vi "Compound_arithmetics.vi"() -> ()   [LabVIEW 2019]
panel:
  in  "num5":dbl
  in  "num4":dbl
  in  "num3":dbl
  in  "num2":dbl
  in  "num1":dbl
  out "result 2":dbl
  in  "E":bool
  in  "D":bool
  in  "C":bool
  in  "B":bool
  out "result":bool
  in  "A":bool
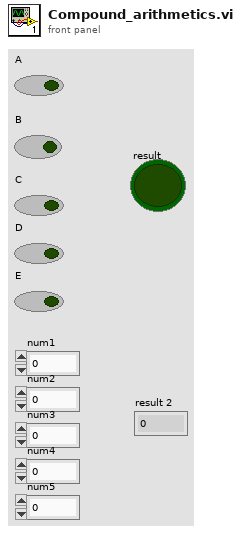
[diagram p1: front panel]
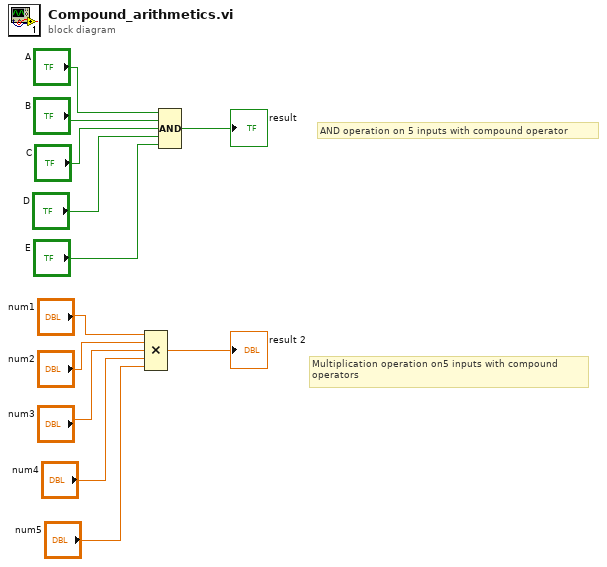
[diagram p0: block diagram]
diagram:
  # "Multiplication operation on5 inputs with compound\noperators"
  # "AND operation on 5 inputs with compound operator"
  n1 = Compound Arithmetic op=MULTIPLY("num1", "num2", "num3", "num4", "num5") -> (→"result 2":dbl)
  n2 = Compound Arithmetic op=AND("A", "B", "C", "D", "E") -> (→"result":bool)
